vi "Example Serial 3.vi"() -> ()   [LabVIEW 2014]
panel:
  out "Error Out":errorcluster
  in  "Error In":errorcluster
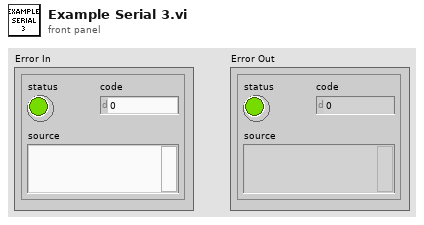
[diagram p1: front panel]
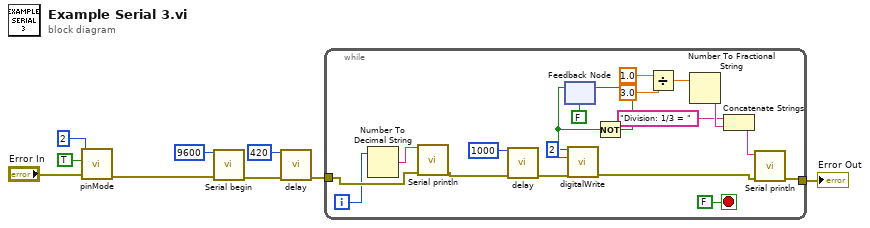
[diagram p0: block diagram]
diagram:
  n1 = call "pinMode.vi"("Error In"="Error In", "output?"=TRUE, "pin number"=2) -> ("Error Out"=w1:errorcluster)  [unwired: 8 in]
  n2 = call "Serial begin.vi"("Error In"=w1, "speed (Bd)"=9600) -> ("Error Out"=w8:errorcluster)  [unwired: 9 in]
  n3 = call "delay.vi"("Error In"=w8, "time (ms)"=420) -> ("Error Out"=w6:errorcluster)  [unwired: 9 in]
  n4 = while {
    tunnel: w6 -> [w26]
    tunnel: [w18] -> w5
    i -> [w14]
    stop <- FALSE stop-if-true
    n5 = Number To Decimal String(number=w14) -> (decimal integer string=w27:string)  [unwired: 1 in]
    n6 = call "Serial println.vi"("Error In"=w26, "string in"=w27) -> ("Error Out"=w24:errorcluster)  [unwired: 9 in]
    n7 = call "delay.vi"("Error In"=w24, "time (ms)"=1000) -> ("Error Out"=w23:errorcluster)  [unwired: 9 in]
    n8 = feedback #1(FALSE) -> (w21:bool)
    n9 = call "digitalWrite.vi"("Error In"=w23, "value"=w21, "pin number"=2) -> ("Error Out"=w17:errorcluster)  [unwired: 8 in]
    n10 = Not(x=w21) -> (.not. x?=w20:bool)
    n11 = feedback-in #1(w20) -> ()
    n12 = Divide(x=1.0, y=3.0) -> (x/y=w15:dbl)
    n13 = Number To Fractional String(number=w15) -> (F-format string=w16:string)  [unwired: 3 in]
    n14 = Concatenate Strings("Division: 1/3 = " ("string"), w16) -> (w10:string)
    n15 = call "Serial println.vi"("Error In"=w17, "string in"=w10) -> ("Error Out"=w18:errorcluster)  [unwired: 9 in]
  }
  "Error Out" <- w5
